vi "append to kpro data array 2016.vi"(0 "Feet of\nStainless to be\nUsed (Count) in":i32, 1 "Up hole Pressure Sensor":dbl format="%.2f", 2 "DHT IK":dbl, 5 "Corrected Array in":dbl[][](array[numeric]), 7 "Aux3/EC":dbl format="%#_13g", 9 "Flow":dbl, 12 "Cluster in":T1, 13 "Downhole Pressure Sensor":dbl format="%#_13g", 14 "Downhole Pressure (V)":dbl) -> (3 "Depth Rate":dbl format="%.2f", 4 "Cluster out 2":T1, 6 "Array Out":dbl[][](array[numeric]), 10 "IK":dbl)   [LabVIEW 2016]
uses:
  controls/Kpro hydraulic measurement cluster.ctl
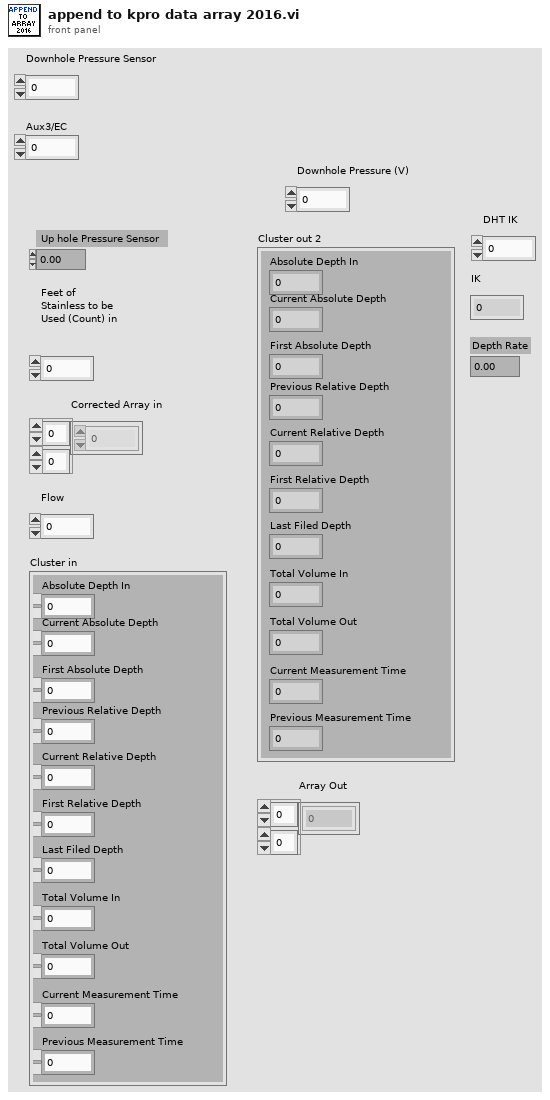
[diagram p1: front panel]
types:
  T1 = typedef "Kpro hydraulic measurement cluster.ctl" = cluster{"Absolute Depth In":dbl, "Current Absolute Depth":dbl, "First Absolute Depth":dbl, "Previous Relative Depth":dbl, "Current Relative Depth":dbl, "First Relative Depth":dbl, "Last Filed Depth":dbl, "Total Volume In":dbl, "Total Volume Out":dbl, "Current Measurement Time":dbl, "Previous Measurement Time":dbl}
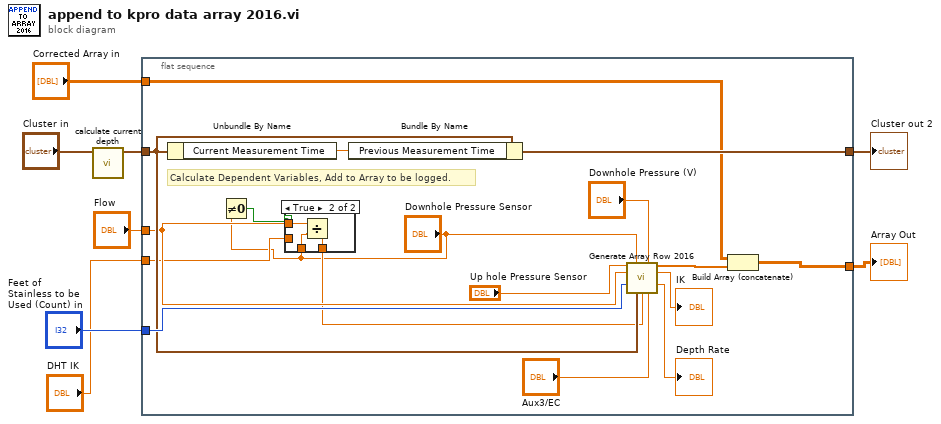
[diagram p0: block diagram]
diagram:
  n1 = call "calculate current depth.vi"("Cluster in"="Cluster in") -> ("Cluster out"=w8:T1)  [unwired: 10 in]
  n2 = flat-sequence {
    tunnel: "Corrected Array in" -> [w16]
    tunnel: "Feet of\nStainless to be\nUsed (Count) in" -> [w25]
    tunnel: "Flow" -> [w13]
    tunnel: w8 -> [w23]
    tunnel: [w21] -> w6
    tunnel: [w17] -> w2
    tunnel: "DHT IK" -> [w11]
    frame #0 {
      # "Calculate Dependent Variables, Add to Array to be logged."
      n3 = Unbundle By Name(w23) -> ("Current Measurement Time"=w22:dbl)
      n4 = Not Equal To 0?(x="Downhole Pressure Sensor") -> (x != 0?=w10:bool)
      n5 = case shown="True" w10 {
        tunnel: w13 -> [_ w29]
        tunnel: "Downhole Pressure Sensor" -> [_ w28]
        tunnel: [w26 w27] -> w12
        tunnel: w11 -> [w26 _]
        frame False {
        }
        frame True {
          n6 = Divide(x=w29, y=w28) -> (x/y=w27:dbl)
        }
      }
      n7 = Bundle By Name(cluster=w23, "Previous Measurement Time"=w22) -> (w21:T1)
      n8 = call "Generate Array Row 2016.vi"("In line Pressure Sensor"="Up hole Pressure Sensor", "Downhole Pressure (ft/H20)"="Downhole Pressure Sensor", "Downhole Pressure (V)"="Downhole Pressure (V)", "Flow"=w13, "Feet of\nStainless to be\nUsed (Count)"=w25, "Cluster"=w23, "DHT IK"=w12, "Aux3/EC"="Aux3/EC") -> ("Array"=w18:dbl[], "IK"=→"IK":dbl, "Depth Rate"=→"Depth Rate":dbl)  [unwired: 5 in]
      n9 = Build Array (concatenate)(w16, w18) -> (w17:dbl[][])
    }
  }
  "Cluster out 2" <- w6
  "Array Out" <- w2
